vi "Station Reference.vi"(8 "error in (no error)":errorcluster, 10 "Action (0: Create)":T1=enum."Set Station Ref", 11 "Station in":refnum<class "Station.lvclass">) -> (0 "error out":errorcluster, 3 "Station out":refnum<class "Station.lvclass">)   [LabVIEW 2018, in "Station.lvclass"]
uses:
  Station.lvclass
  Controls/Server Control.ctl
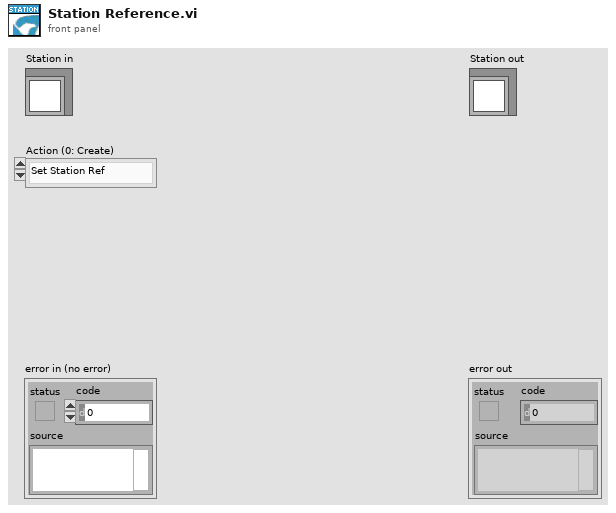
[diagram p1: front panel]
types:
  T1 = typedef "Server Control.ctl" = enum16{"Open New Reference", "Remove Reference", "Kill Server", "Set Station Ref", "Get Station Ref"}
  T2 = cluster{"Action (0: Create)":T1, path, "Station in":refnum<class "Station.lvclass">}
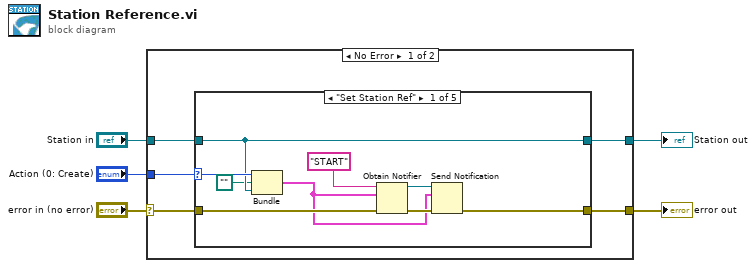
[diagram p0: block diagram]
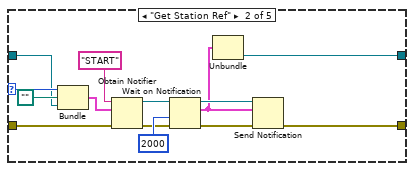
[diagram p2: hidden frame]
diagram:
  n1 = case shown="No Error" "error in (no error)" {
    selector: "error in (no error)" -> [w8 w41]
    tunnel: [w7 w41] -> w4
    tunnel: [w6 w40] -> w2
    tunnel: "Station in" -> [w9 w40]
    tunnel: "Action (0: Create)" -> [w10 _]
    frame No Error {
      n2 = case shown="\"Set Station Ref\"" w10 {
        selector: w10 -> [w19 w33 _ _ _]
        tunnel: w9 -> [w17 w29 w35 w37 w39]
        tunnel: w8 -> [w18 w32 w34 w36 w38]
        tunnel: [w13 w22 w34 w36 w38] -> w7
        tunnel: [w17 w28 w35 w37 w39] -> w6
        frame "Set Station Ref" {
          n3 = Bundle("Action (0: Create)"=w19, path "", "Station in"=w17) -> (w11:T2)  [unwired: 1 in]
          n4 = Obtain Notifier(name (unnamed)="START", notification data type=w11, error in (no error)=w18) -> (notifier out=w14:refnum<notifier>, error out=w15:errorcluster)  [unwired: 1 in, 1 out]
          n5 = Send Notification(notification=w11, notifier=w14, error in (no error)=w15) -> (error out=w13:errorcluster)  [unwired: 1 out]
        }
        frame "Get Station Ref" {
          n6 = Bundle("Action (0: Create)"=w33, path "", "Station in"=w29) -> (w25:T2)  [unwired: 1 in]
          n7 = Obtain Notifier(name (unnamed)="START", notification data type=w25, error in (no error)=w32) -> (notifier out=w27:refnum<notifier>, error out=w26:errorcluster)  [unwired: 1 in, 1 out]
          n8 = Wait on Notification(notifier=w27, timeout in ms (-1)=2000, error in (no error)=w26) -> (notifier out=w21:refnum<notifier>, notification=w20:T2, error out=w23:errorcluster)  [unwired: 1 in, 1 out]
          n9 = Unbundle(w20) -> ("Station in"=w28:refnum<class "Station.lvclass">)  [unwired: 2 out]
          n10 = Send Notification(notification=w20, notifier=w21, error in (no error)=w23) -> (error out=w22:errorcluster)  [unwired: 1 out]
        }
        frame "Kill Server" {
        }
        frame "Remove Reference" {
        }
        frame "Open New Reference" {
        }
      }
    }
    frame Error {
    }
  }
  "error out" <- w4
  "Station out" <- w2
